vi "获取简易流程列表.vi"(8 "error in (no error)":errorcluster, 10 "添加的路径":path, 11 "查询参数":string) -> (0 "error out":errorcluster, 3 "简易流程列表":cluster{"String":string, "Value":u16}[](array[cluster]))   [LabVIEW 2022 SP3, in "Cleaning cycle.lvclass"]
uses:
  Cleaning cycle.lvclass
  <vilib>/xml/Load XML File.vi
  <vilib>/xml/Close Reference(Node).vi
  <vilib>/xml/NI_XML.lvlib
  <resource>/objmgr/DOMUserDefRef.rc
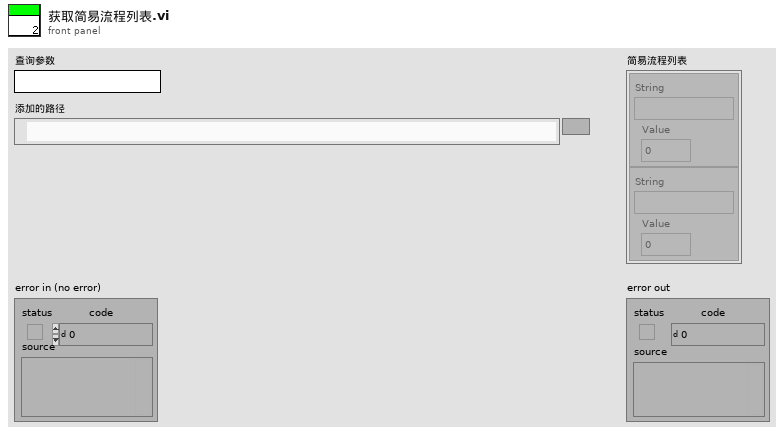
[diagram p1: front panel]
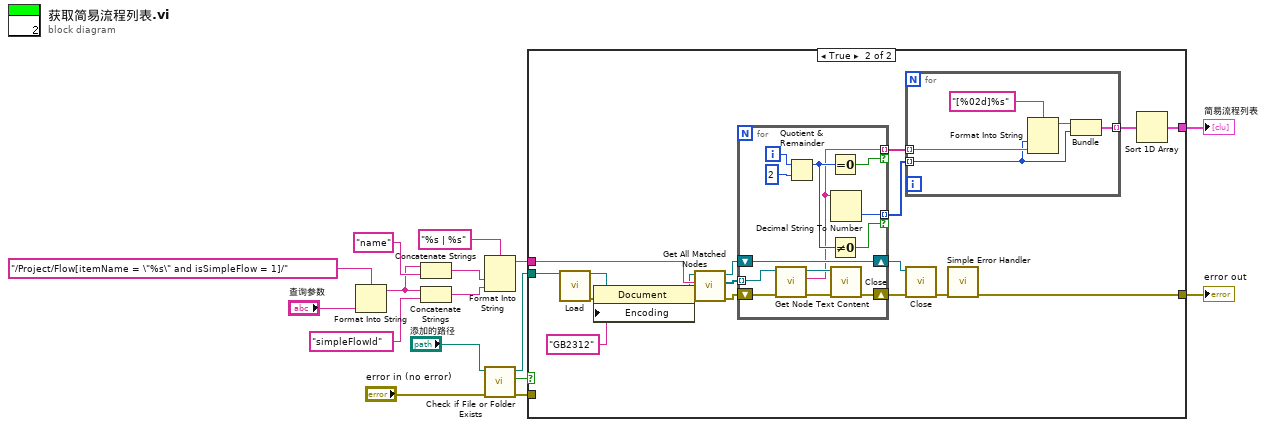
[diagram p0: block diagram]
diagram:
  n1 = Format Into String(format string="/Project/Flow[itemName = \"%s\" and isSimpleFlow = 1]/" ("格式字符串"), "查询参数") -> (resulting string=w13:string)  [unwired: 2 in, 1 out]
  n2 = Concatenate Strings(w13, "name" ("字符串")) -> (w10:string)
  n3 = Concatenate Strings(w13, "simpleFlowId" ("字符串")) -> (w9:string)
  n4 = Format Into String(format string="%s | %s" ("格式字符串"), w10, w9) -> (resulting string=w4:string)  [unwired: 2 in, 1 out]
  n5 = call <vilib>:"Check if File or Folder Exists.vi"("error in (no error)"="error in (no error)", "path"="添加的路径") -> ("error out"=w5:errorcluster, "file or folder exists?"=w6:bool, "dup path"=w7:path)  [unwired: 7 in]
  n6 = case shown="True" w6 {
    tunnel: w7 -> [_ w34]
    tunnel: w4 -> [_ w27]
    tunnel: w5 -> [_ _]
    tunnel: [_ w19] -> w2
    tunnel: [_ w17] -> w1
    frame False {
    }
    frame True {
      n7 = call-poly <vilib>:"Load.vi"("path to XML document"=w34) -> ("DOM document out"=w31:refnum<k20>, "error out"=w30:errorcluster)  [unwired: 12 in, 1 out]
      n8 = property on="属性节点" class="Document"(reference=w31, error in=w30, "Encoding"="GB2312" ("文档编码")) -> (reference out=w25:refnum<k20>, error out=w24:errorcluster)
      n9 = call <vilib>:"Get All Matched Nodes.vi"("error in (no error)"=w24, "XPath expression"=w27, "node in"=w25) -> ("error out"=w28:errorcluster, "node result array"=w29:refnum<k20>[], "node out"=w23:refnum<k20>)  [unwired: 6 in]
      n10 = for {
        tunnel: w29 -> [w48] mode=indexing
        shift-right: [w49] -> w26
        shift-left: w28 -> [w52]
        shift-right: [w47] -> w22
        shift-left: w23 -> [w47]
        tunnel: [w40] -> w21 mode=indexing if=w44
        tunnel: [w41] -> w20 mode=indexing if=w42
        i -> [w46]
        n11 = call <vilib>:"Get Node Text Content.vi"("error in (no error)"=w52, "node in"=w48) -> ("error out"=w50:errorcluster, "node text"=w40:string, "node out"=w51:refnum<k20>)  [unwired: 7 in]
        n12 = Quotient & Remainder(x=w46, y=2) -> (x-y*floor(x/y)=w43:i32)  [unwired: 1 out]
        n13 = Equal To 0?(x=w43) -> (x = 0?=w44:bool)
        n14 = Not Equal To 0?(x=w43) -> (x != 0?=w42:bool)
        n15 = Decimal String To Number(string=w40) -> (number=w41:i32)  [unwired: 2 in, 1 out]
        n16 = call-poly <vilib>:"Close.vi"("error in (no error)"=w50, "node"=w51) -> ("error out"=w49:errorcluster)  [unwired: 7 out]
      }
      n17 = for {
        tunnel: w21 -> [w38] mode=indexing
        tunnel: w20 -> [w36] mode=indexing
        tunnel: [w35] -> w18 mode=indexing
        n18 = Format Into String(format string="[%02d]%s" ("格式字符串"), w36, w38) -> (resulting string=w37:string)  [unwired: 2 in, 1 out]
        n19 = Bundle(w37, w36) -> (w35:cluster{string, i32})  [unwired: 1 in]
      }
      n20 = call-poly <vilib>:"Close.vi"("error in (no error)"=w26, "node"=w22) -> ("error out"=w33:errorcluster)  [unwired: 7 out]
      n21 = call <vilib>:"Simple Error Handler.vi"("error in (no error)"=w33) -> ("error out"=w19:errorcluster)  [unwired: 4 in, 4 out]
      n22 = Sort 1D Array(array=w18) -> (sorted array=w17:cluster{string, i32}[])
    }
  }
  "简易流程列表" <- w1
  "error out" <- w2
